vi "strobe.vi"() -> ()   [LabVIEW 2012]
uses:
  <vilib>/Platform/TimedLoop/XDataNode/timing_clust.ctl
  <vilib>/Platform/TimedLoop/XDataNode/nitl_modes.ctl
  <vilib>/Platform/TimedLoop/XDataNode/wakeup.ctl
  initialization/micron_globals.vi
  <vilib>/DAQmx/create/channels.llb/DAQmx Create Channel (CO-Pulse Generation-Frequency).vi
  <vilib>/DAQmx/configure/timing.llb/DAQmx Timing (Implicit).vi
  <vilib>/Platform/TimedLoop/XDataNode/XDataNode.xnode
  <resource>/objmgr/daqmx.rc
  <vilib>/Platform/TimedLoop/XDataNode/XDNodeRunTimeDep.lvlib
panel:
  out "Sweep duration":dbl min=0.0 step=0.001 format="%#_3p"
  out "Running":bool
  in  "Arm":bool
  out "Task":refnum<k21>
  out "Pulse rate":dbl
  in  "stop":bool
  out "Time":dbl min=0.0 step=0.001 format="%#_5p"
  in  "Offset":dbl(slide)=0.5 step=0.2 scale=-2.0..2.0 scale format="%#_2g"
  out "Phase":dbl step=5.0 format="%#.1f"
  out "Period":dbl min=0.0 step=0.001 format="%#_5p"
  in  "Center frequency":dbl(slide)=1.0 min=0.0 max=10000.0 step=1.0 scale=10.0..500.0 scale format="%#_5p"
  out "Length":dbl min=0.0 step=0.001 format="%#_5p"
  in  "Duty cycle":dbl(slide)=0.003390806681894051 scale=0.0001..0.1 scale format="%#_2g"
  in  "Sweep":cluster{"Phase":dbl, "Time":dbl}[](array[cluster])=[{"Phase"=0.0, "Time"=0.0}, {"Phase"=0.0, "Time"=0.0}] {"Time" min=0.0 step=0.001 format="%#_4p"; "Phase" step=5.0 format="%#.0f"}
  in  "Mode":bool
  in  "Source":enum16{"Auto", "Manual", "Fs"}(ring)
  # "Strobe controller"
  # "Phase"
  # "Time"
  # "Frequency"
  # "Start"
  # "End"
  # "Triggered"
  # "Continuous"
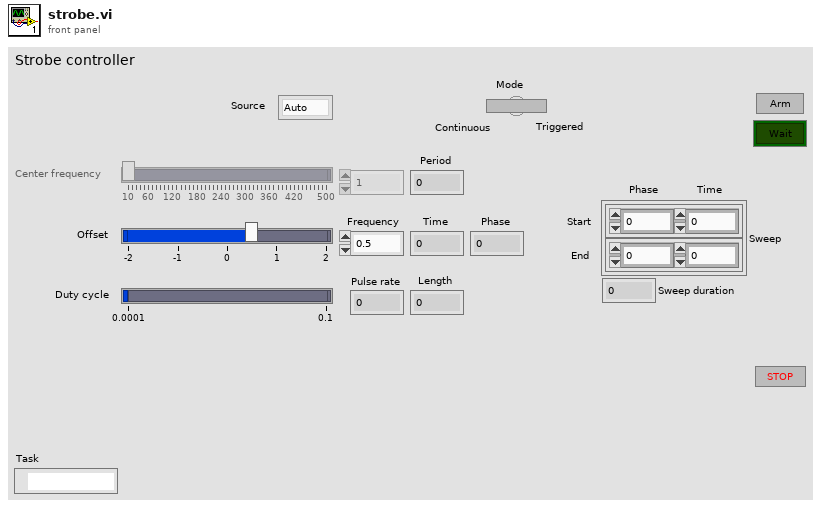
[diagram p1: front panel]
types:
  T1 = cluster{"Pulse rate":dbl, "Duty cycle":dbl, "Time":dbl, "f":i32}
  T2 = typedef "XDNodeRunTimeDep.lvlib/timing_clust.ctl" = cluster{"Expected End [f-1]":u64, "Actual End [f-1]":u64, "Finished Late? [f-1]":bool, "Expected End [i-1]":u64, "Actual End [i-1]":u64, "Finished Late? [i-1]":bool, "Expected Start [i]":u64, "Actual Start [i]":u64, "Expected Start [f]":u64, "Actual Start [f]":u64, "Source Name":string, "Structure Name":string, "Period":i64, "Deadline":i64, "Offset":i64, "Start":i64, "Priority":i32, "Timeout":i32, "Mode":T3, "Wakeup Reason":T4, "Error":errorcluster, "Source Type":string, "Secondary Source Type":string, "Global End Time":u64, "Global Start Time":u64, "Frame Duration":u64, "Iteration Duration":u64, "Assigned CPU":i32, "I/O Scan Engine Mode":u32}
  T3 = typedef "XDNodeRunTimeDep.lvlib/nitl_modes.ctl" = enum32{"No Change", "Process missed periods, maintain original phase", "Discard missed periods, maintain original phase", "Process missed periods, ignore original phase", "Discard missed periods, ignore original phase"}
  T4 = typedef "XDNodeRunTimeDep.lvlib/wakeup.ctl" = enum32{"Normal", "Aborted", "Asynchronous wakeup", "Timing source error", "Timed loop error", "Timeout"}
  T5 = typedef "micron_config.ctl" = cluster{"rt fifo":refnum<k33>, "Analog output task":refnum<k21>, "Analog output task 2":refnum<k21>, "Stimulus AO task":refnum<k21>, "Low-rate AIN task":refnum<k21>, "Pedal out task":refnum<k21>, "Pedal in task":refnum<k21>, "Loop timing source":string, "Relay out task":refnum<k21>, "Send UDP Conn":refnum<k16>, "Recv UDP Conn":refnum<k16>, "Host Addr":dbl, "I2C interface":T6, "trace_start notifier":refnum<notifier>, "trace_done notifier":refnum<notifier>, "ASAP FIFO":refnum<k33>}
  T6 = typedef "i2c_interface.ctl" = cluster{"FPGA VI Reference":T7}
  T7 = typedef "fpga_reference.ctl" = refnum<k20>
  T8 = enum8{"Enabled", "Disabled", "Disabled and Grayed Out"}
  T9 = typedef "Micron params.ctl" = cluster{"Stimulus":T10, "Goal Filter A":T12, "Mode controls":T13, "Manipulator type":enum16{"Current piezo", "Voltage piezo"}, "Manipulator calibration":T14, "Network":T16, "Goal Filter B":T12, "Cancellation":T17, "Transition time":sgl, "Estimation":T19}
  T10 = typedef "stimulus.ctl" = cluster{"Type":enum16{"Off", "Step", "Sine", "Triangle", "Arbitrary"}, "Phase":dbl, "Amplitude":sgl[], "Injection point":T11, "Closed loop":bool, "Offset":sgl[], "Tip -> world":bool, "Frequency":dbl, "Length":dbl}
  T11 = typedef "injection_point.ctl" = enum16{"Total pose", "V limiter", "Goal ", "Link position", "KF link position", "Link goal", "Link error", "Controller", "Output", "Drive", "Light"}
  T12 = typedef "goal_loop_parms.ctl" = cluster{"Speedup max":sgl, "Speedup thresh":sgl, "Speedup nonlin":sgl, "Filters":cluster{"Lower Fc":sgl, "Lower Q":sgl, "Scale factor":sgl, "Upper Fc":sgl, "Upper Q":sgl, "V limit":sgl, "V limit range":sgl}[]}
  T13 = typedef "mode_conrols.ctl" = cluster{"Hold":bool, "Cancellation":bool, "Goal filter":bool, "Trigger":bool}
  T14 = typedef "manipulator_cal.ctl" = cluster{"Tool offsets":sgl[][], "Tip light calibration":T15, "Handle light calibration":T15, "Base pivots":sgl[][], "Output pivots":sgl[][], "Length center":sgl, "Workspace height":sgl[], "Workspace diameter":sgl[], "Linearization":sgl[][], "Stack travel":sgl, "Saturation pos":sgl, "Inverse filters":cluster{"filter structure":enum32{"IIR 2nd Order", "IIR 4th Order"}, "Reverse Coefficients":dbl[], "Forward Coefficients":dbl[]}[]}
  T15 = typedef "probe_calibration.ctl" = sgl[][]
  T16 = typedef "network_params.ctl" = cluster{"Remote Host":string, "Send Status":bool, "Send Port":u16, "Recv Commands":bool, "Recv Port":u16}
  T17 = typedef "sq_control_params.ctl" = cluster{"KP":T18, "KI":sgl, "KD":T18, "Max vel":sgl, "Max acc":sgl, "Int error limit":sgl, "RCM gain":sgl, "Bypass":bool, "Degraded gain":sgl}
  T18 = typedef "decoupled_gain.ctl" = cluster{"XY":sgl, "Rxy":sgl, "Z":sgl, "Rz":sgl}
  T19 = typedef "estimation_controls.ctl" = cluster{"Link":cluster{"Measure noise":dbl[], "Process noise":dbl[], "Alt process noise":dbl[], "Innovation limit":dbl[], "Residue threshold":dbl, "Enable":bool}, "Handle":cluster{"Measure noise":dbl[], "Process noise":dbl[], "State limits":dbl[], "Innovation limit":dbl[], "Prediction Lookahead":sgl, "Enable":bool}}
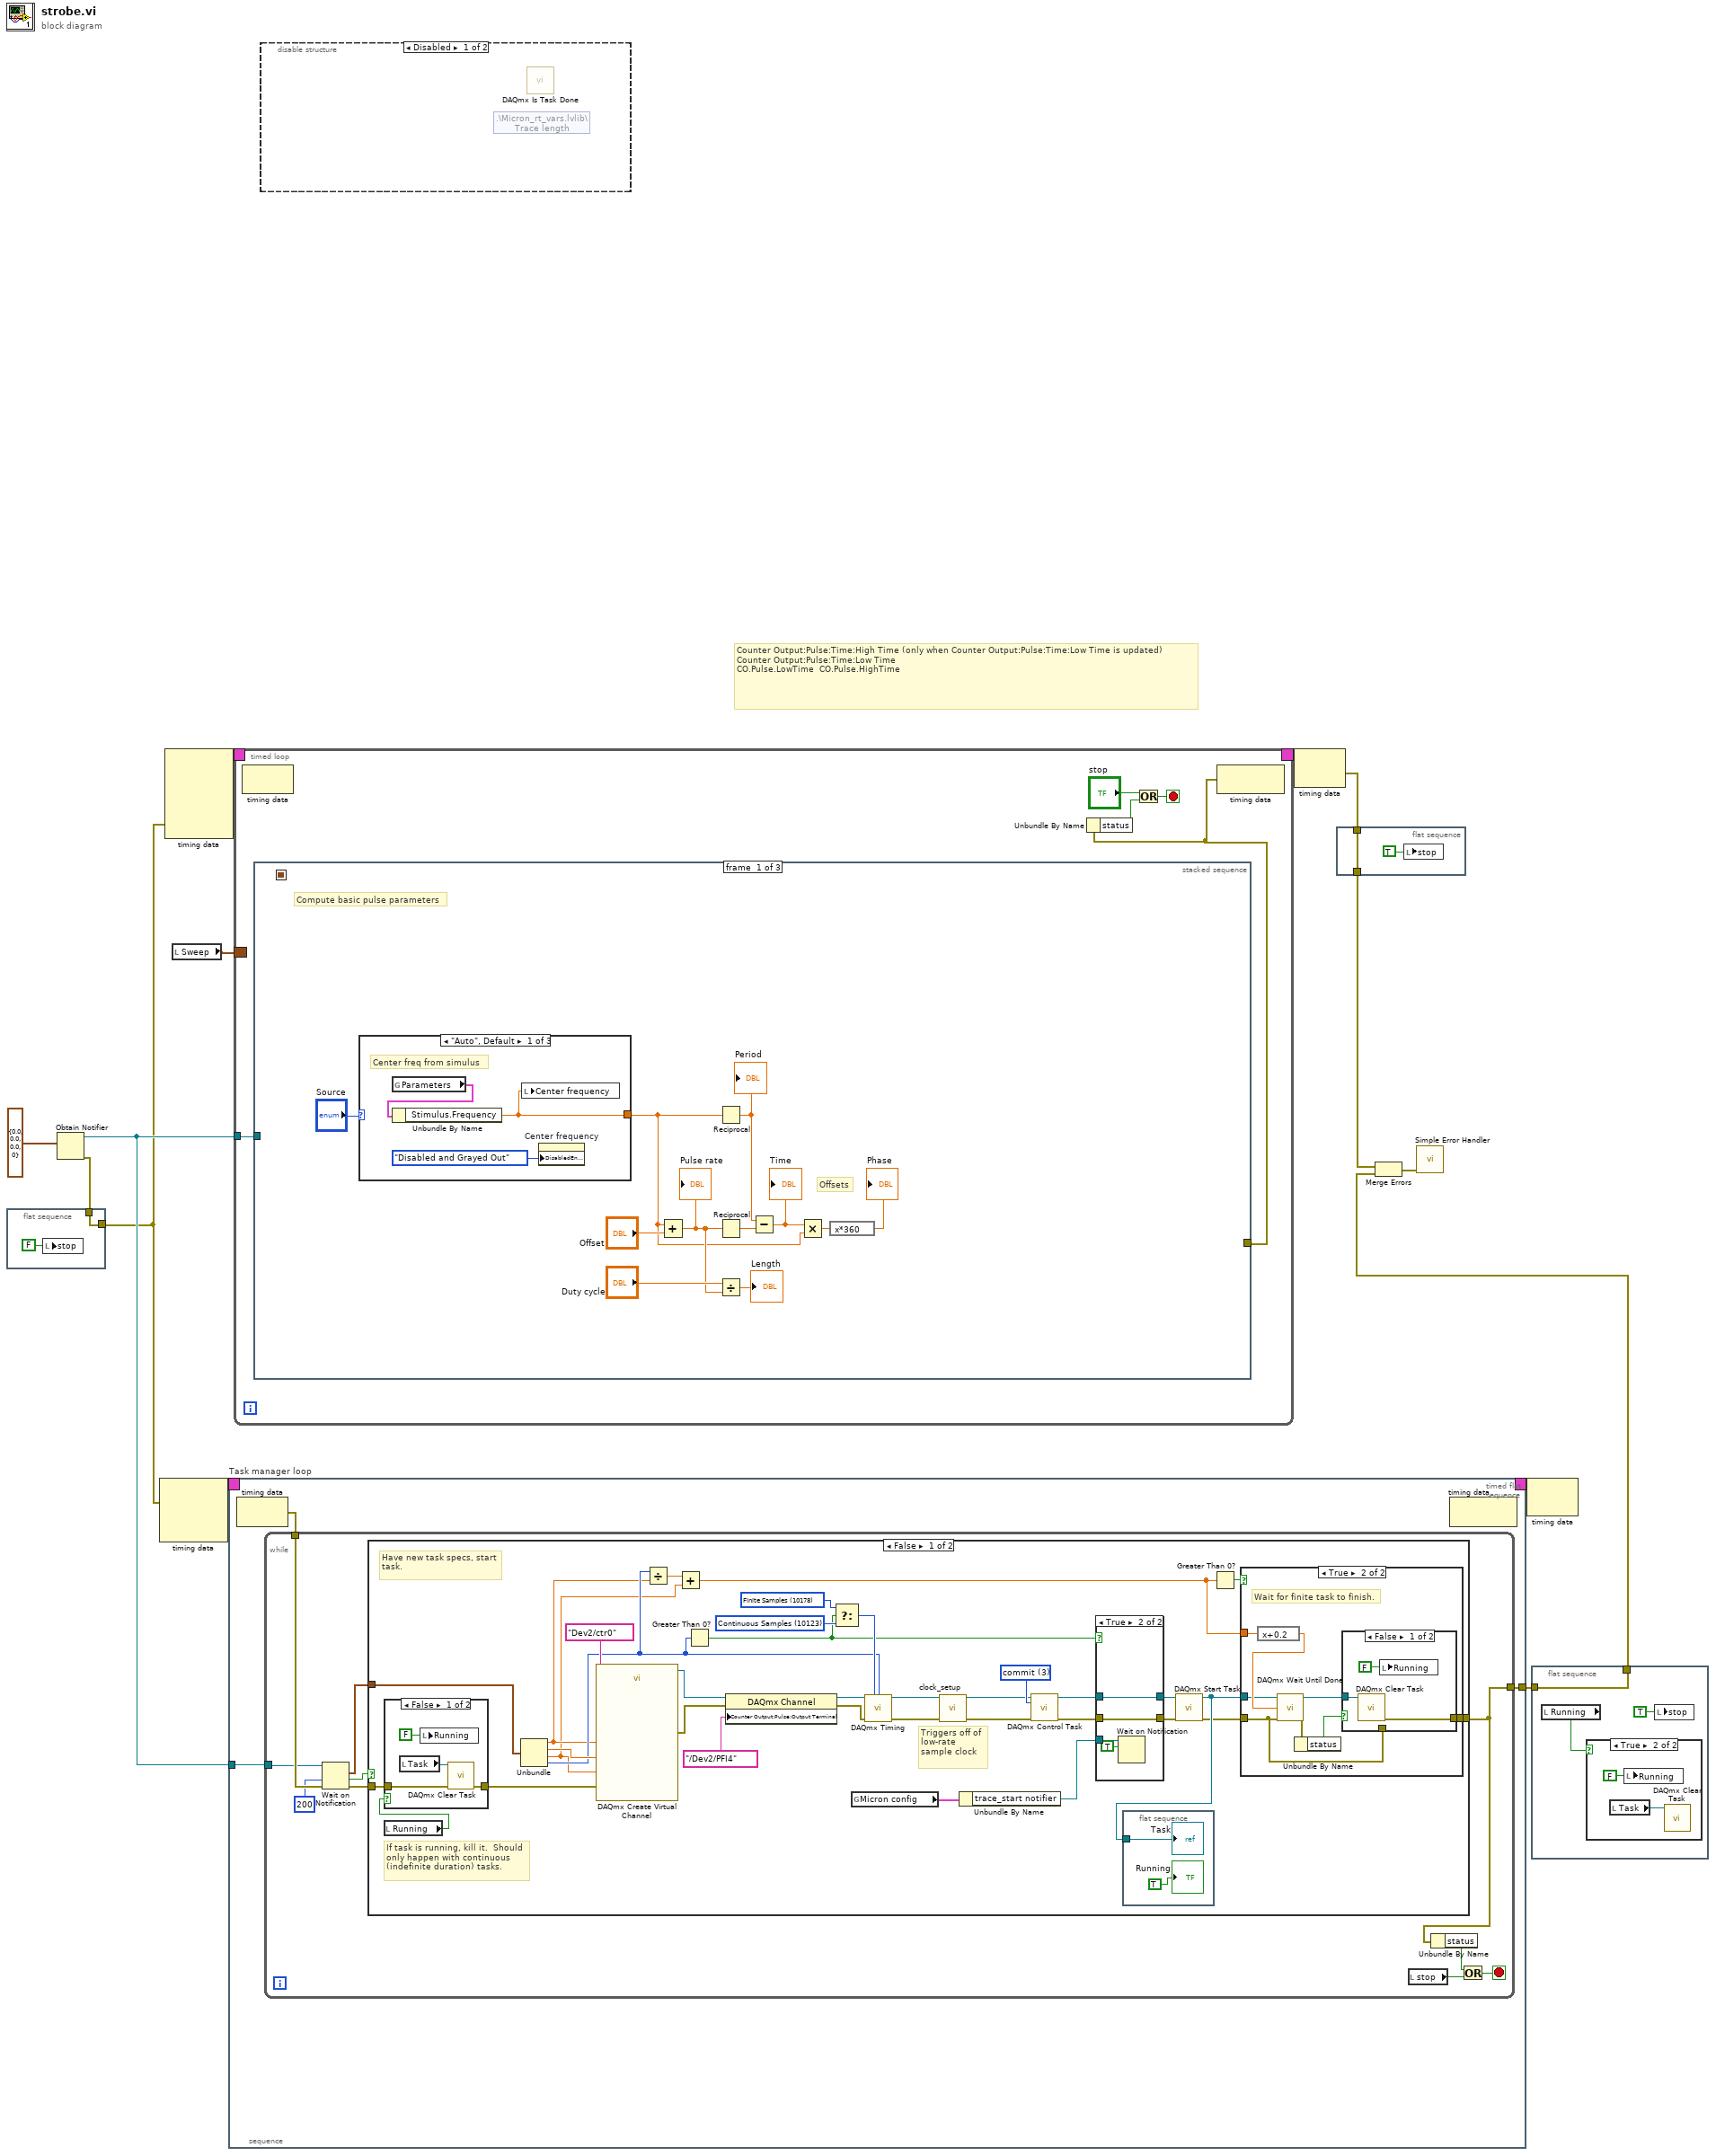
[diagram p0: block diagram]
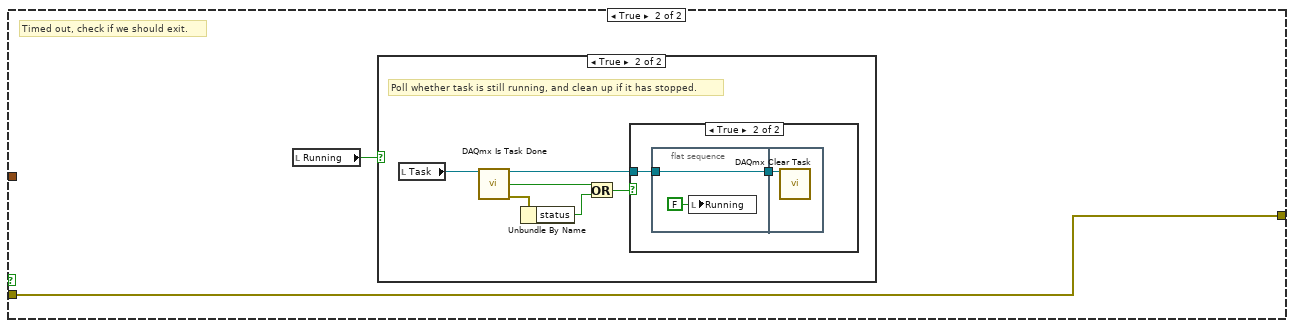
[diagram p7: hidden frame]
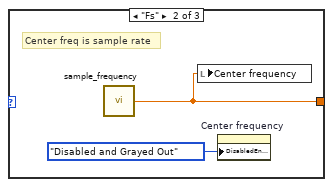
[diagram p10: hidden frame]
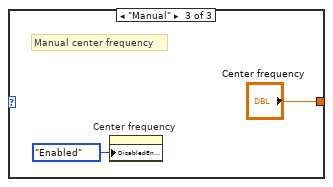
[diagram p11: hidden frame]
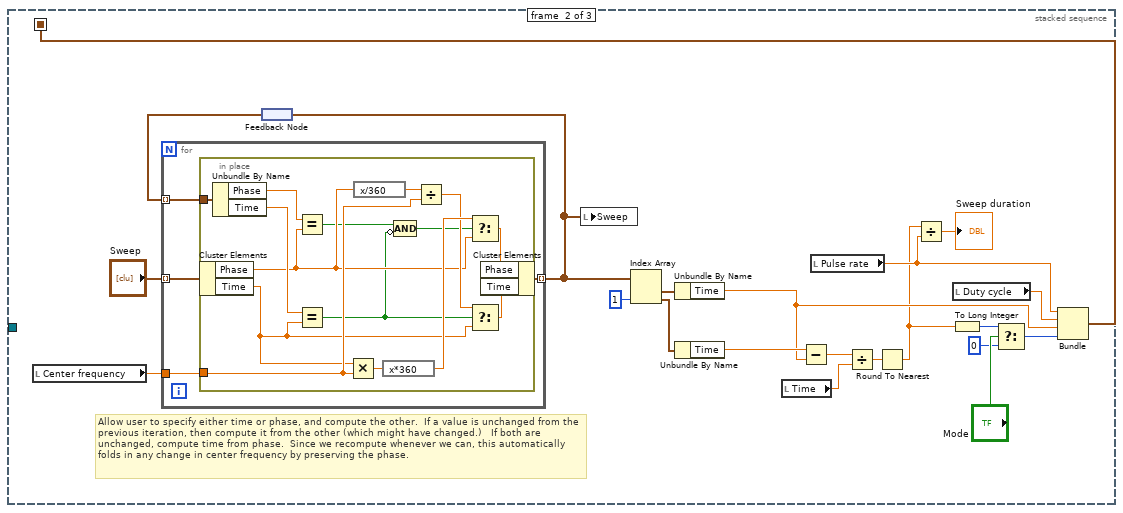
[diagram p12: hidden frame]
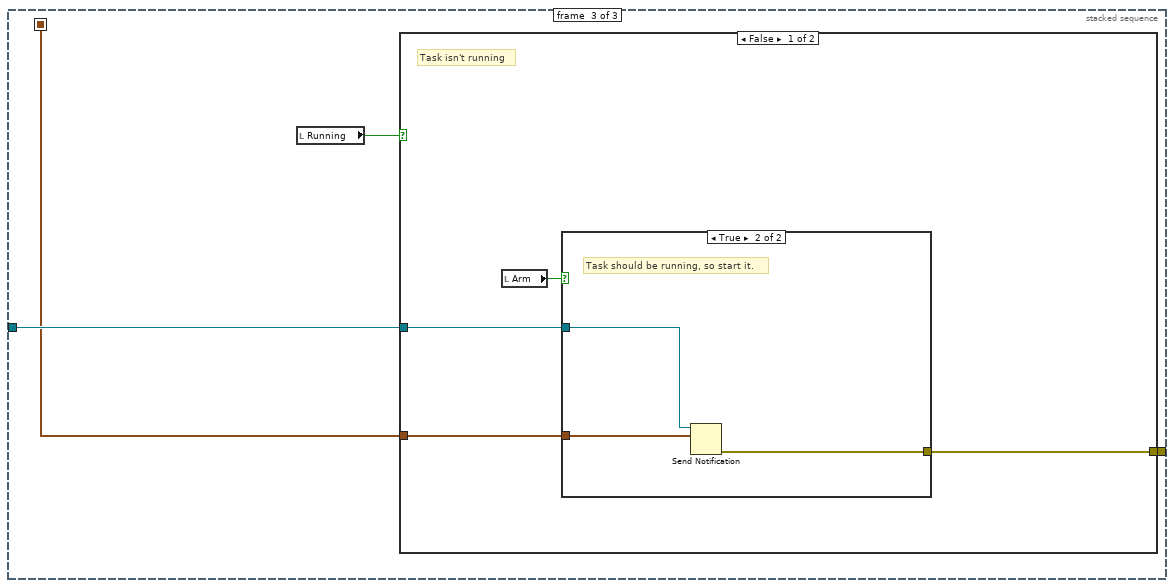
[diagram p13: hidden frame]
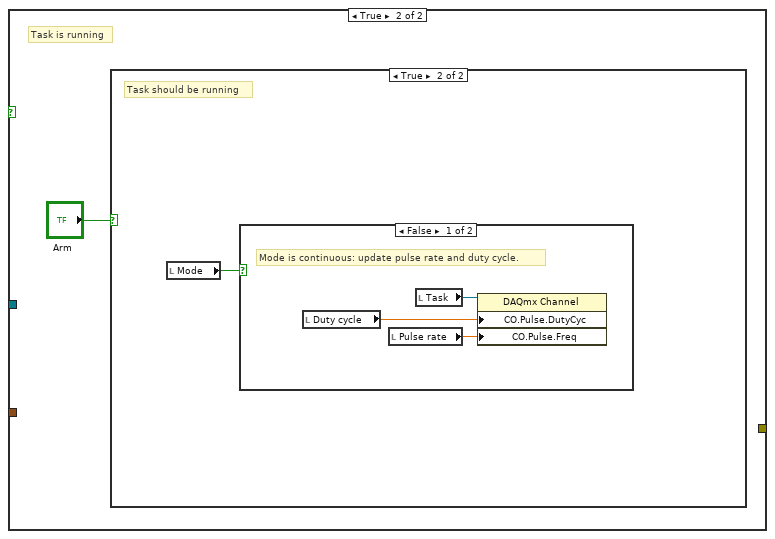
[diagram p15: hidden frame]
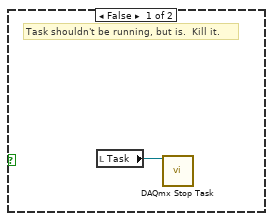
[diagram p16: hidden frame]
diagram:
  # "Counter Output:Pulse:Time:High Time (only when Counter Output:Pulse:Time:Low Time is updated) \nCounter Output:Pulse:Time:Low Time\nCO.Pulse.LowTime  CO.Pulse.HighTime"
  n1 = flat-sequence {
    tunnel: w8 -> [w16]
    tunnel: [w16] -> w7
    frame #0 {
      n2 = local write "stop"(FALSE ("stop")) -> ()
    }
  }
  n3 = Obtain Notifier(notification data type=T1 {"Pulse rate"=0.0, "Duty cycle"=0.0, "Time"=0.0, "f"=0} ("output cluster")) -> (notifier out=w10:refnum<notifier>, error out=w8:errorcluster)  [unwired: 3 in, 1 out]
  n4 = node-c288(w7) -> (w12:T2)  [unwired: 2 in]
  n5 = node-c288(w7) -> (w14:T2)  [unwired: 4 in]
  n6 = local read "Sweep"() -> (w1:cluster{"Phase":dbl, "Time":dbl}[])
  n7 = timed-sequence "Task manager loop" {
    timing: w12 -> [_]
    timing-out: [_] -> w11
    tunnel: w10 -> [w18]
    tunnel: [w17] -> w2
    n8 = timed-flat-sequence {
      tunnel: w18 -> [w20]
      tunnel: [w19] -> w17
      n9 = node-c288() -> (w21:errorcluster)  [unwired: 1 in]
      n10 = while {
        tunnel: w21 -> [w31]
        tunnel: w20 -> [w30]
        tunnel: [w22] -> w19
        stop <- w25 stop-if-true
        n11 = Wait on Notification(notifier=w30, timeout in ms (-1)=200, error in (no error)=w31) -> (notification=w29:T1, timed out?=w24:bool, error out=w28:errorcluster)  [unwired: 1 in, 1 out]
        n12 = case shown="False" w24 {
          tunnel: w29 -> [w53 _]
          tunnel: w28 -> [w41 w94]
          tunnel: [w35 w94] -> w22
          frame False {
            w50 = 10123 items=["Finite Samples"=10178, "Continuous Samples"=10123, "Hardware Timed Single Point"=12522] ("sample mode")
            w51 = 10178 items=["Finite Samples"=10178, "Continuous Samples"=10123, "Hardware Timed Single Point"=12522] ("sample mode")
            w62 = 3 items=["verify"=2, "reserve"=4, "commit"=3, "unreserve"=5, "abort"=6] ("action")
            # "If task is running, kill it.  Should\nonly happen with continuous\n(indefinite duration) tasks."
            # "Have new task specs, start task."
            # "Triggers off of low-rate sample clock"
            n13 = local read "Running"() -> (w39:bool)
            n14 = case shown="False" w39 {
              tunnel: [w85 w86] -> w40
              tunnel: w41 -> [w82 w86]
              frame False {
                n15 = local read "Task"() -> (w83:refnum<k21>)
                n16 = local write "Running"(FALSE ("Running")) -> ()
                n17 = call <vilib>:"DAQmx Clear Task.vi"("task in"=w83, "error in"=w82) -> ("error out"=w85:errorcluster)  [unwired: 13 in]
              }
              frame True {
              }
            }
            n18 = Unbundle(w53) -> ("Pulse rate"=w42:dbl, "Duty cycle"=w52:dbl, "Time"=w32:dbl, "f"=w43:i32)
            n19 = call-poly <vilib>:"DAQmx Create Virtual Channel.vi"("frequency"=w42, "duty cycle"=w52, "counter"=tag "Dev2/ctr0" ("Counter(s)"), "error in"=w40, "initial delay"=w32) -> ("task out"=w58:refnum<k21>, "error out"=w57:errorcluster)  [unwired: 4 in, 5 out]
            n20 = Divide(x=w43, y=w42) -> (x/y=w34:dbl)
            n21 = Add(x=w34, y=w32) -> (x+y=w33:dbl)
            n22 = Greater Than 0?(x=w43) -> (x > 0?=w46:bool)
            n23 = property class="DAQmx Channel"(reference=w58, error in=w57, "Counter Output:Pulse:Output Terminal"=tag "/Dev2/PFI4" ("CO.Pulse.Term")) -> (reference out=w56:refnum<k21>, error out=w55:errorcluster)
            n24 = Select(t=w51, s=w46, f=w50) -> (s? t:f=w49:i32)
            n25 = global read "micron_globals.vi" "Micron config"() -> (w45:T5)
            n26 = call-poly <vilib>:"DAQmx Timing.vi"("task/channels in"=w56, "sample mode"=w49, "samples per channel"=w43, "error in"=w55) -> ("task out"=w61:refnum<k21>, "error out"=w60:errorcluster)  [unwired: 10 out]
            n27 = call "clock_setup.vi"("task in"=w61, "error in"=w60) -> ("task out"=w48:refnum<k21>, "error out"=w47:errorcluster)  [unwired: 12 in]
            n28 = Unbundle By Name(w45) -> ("trace_start notifier"=w44:refnum<notifier>)
            n29 = call <vilib>:"DAQmx Control Task.vi"("task/channels in"=w48, "action"=w62, "error in"=w47) -> ("task out"=w65:refnum<k21>, "error out"=w63:errorcluster)  [unwired: 11 in]
            n30 = case shown="True" w46 {
              tunnel: w63 -> [w87 w92]
              tunnel: [w87 w92] -> w64
              tunnel: w65 -> [w88 w91]
              tunnel: [w88 w91] -> w66
              tunnel: w44 -> [_ w90]
              frame False {
              }
              frame True {
                n31 = Wait on Notification(notifier=w90, ignore previous (F)=TRUE) -> ()  [unwired: 2 in, 4 out]
              }
            }
            n32 = flat-sequence {
              tunnel: w37 -> [w80]
              frame #0 {
                "Task" <- w80
                "Running" <- TRUE ("Running")
              }
            }
            n33 = call <vilib>:"DAQmx Start Task.vi"("task/channels in"=w66, "error in"=w64) -> ("task out"=w37:refnum<k21>, "error out"=w36:errorcluster)  [unwired: 12 in]
            n34 = Greater Than 0?(x=w33) -> (x > 0?=w38:bool)
            n35 = case shown="True" w38 {
              tunnel: w33 -> [_ w74]
              tunnel: w37 -> [_ w72]
              tunnel: w36 -> [w67 w68]
              tunnel: [w67 w69] -> w35
              frame False {
              }
              frame True {
                # "Wait for finite task to finish."
                n36 = expression code="x+0.2"(w74) -> (w73:dbl)
                n37 = call <vilib>:"DAQmx Wait Until Done.vi"("task/channels in"=w72, "timeout (sec)"=w73, "error in"=w68) -> ("task out"=w75:refnum<k21>, "error out"=w71:errorcluster)  [unwired: 11 in]
                n38 = Unbundle By Name(w71) -> ("status"=w70:bool)
                n39 = case shown="False" w70 {
                  tunnel: w75 -> [w78 _]
                  tunnel: [w77 w79] -> w69
                  tunnel: w68 -> [_ w79]
                  frame False {
                    n40 = call <vilib>:"DAQmx Clear Task.vi"("task in"=w78) -> ("error out"=w77:errorcluster)  [unwired: 14 in]
                    n41 = local write "Running"(FALSE ("Running")) -> ()
                  }
                  frame True {
                  }
                }
              }
            }
          }
          frame True {
            # "Timed out, check if we should exit."
            n42 = local read "Running"() -> (w93:bool)
            n43 = case shown="True" w93 {
              frame False {
              }
              frame True {
                # "Poll whether task is still running, and clean up if it has stopped."
                n44 = local read "Task"() -> (w100:refnum<k21>)
                n45 = call <vilib>:"DAQmx Is Task Done.vi"("task/channels in"=w100) -> ("task out"=w95:refnum<k21>, "task done?"=w97:bool, "error out"=w99:errorcluster)  [unwired: 12 in]
                n46 = Unbundle By Name(w99) -> ("status"=w98:bool)
                n47 = Or(x=w97, y=w98) -> (x .or. y?=w96:bool)
                n48 = case shown="True" w96 {
                  tunnel: w95 -> [_ w102]
                  frame False {
                  }
                  frame True {
                    n49 = flat-sequence {
                      tunnel: w102 -> [w104]
                      tunnel: [w104] -> w101
                      tunnel: w101 -> [w105]
                      frame #0 {
                        n50 = local write "Running"(FALSE ("Running")) -> ()
                      }
                      frame #1 {
                        n51 = call <vilib>:"DAQmx Clear Task.vi"("task in"=w105) -> ()  [unwired: 14 in, 1 out]
                      }
                    }
                  }
                }
              }
            }
          }
        }
        n52 = local read "stop"() -> (w27:bool)
        n53 = Unbundle By Name(w22) -> ("status"=w26:bool)
        n54 = Or(x=w26, y=w27) -> (x .or. y?=w25:bool)
      }
      n55 = node-c288() -> ()  [unwired: 1 in, 1 out]
    }
  }
  n56 = timed-loop {
    timing: w14 -> [_]
    timing-out: [_] -> w13
    tunnel: w10 -> [w110]
    border: w1 -> [_]
    stop <- w111 stop-if-true
    n57 = node-c288() -> ()  [unwired: 1 in, 1 out]
    n58 = stacked-sequence {
      seq-local: [_ w136 _] -> [_ _ w177]
      tunnel: [_ _ w179] -> w109
      tunnel: w110 -> [_ _ w178]
      frame #0 {
        # "Compute basic pulse parameters"
        # "Offsets"
        n59 = case shown="\"Auto\", Default" "Source" {
          tunnel: [w129 w132 "Center frequency"] -> w120
          frame "Auto", Default {
            # "Center freq from simulus"
            n60 = global read "micron_globals.vi" "Parameters"() -> (w131:T9)
            n61 = Unbundle By Name(w131) -> ("Stimulus.Frequency"=w129:dbl)
            n62 = local write "Center frequency"(w129) -> ()
            n63 = property on="Center frequency" class="Slide (strict)"("DisabledEnum"=T8."Disabled and Grayed Out" ("Disabled")) -> ()  [unwired: 2 in, 2 out]
          }
          frame "Fs" {
            # "Center freq is sample rate"
            n64 = call "sample_frequency.vi"() -> ("Sample frequency"=w132:dbl)
            n65 = local write "Center frequency"(w132) -> ()
            n66 = property on="Center frequency" class="Slide (strict)"("DisabledEnum"=T8."Disabled and Grayed Out" ("Disabled")) -> ()  [unwired: 2 in, 2 out]
          }
          frame "Manual" {
            # "Manual center frequency"
            n67 = property on="Center frequency" class="Slide (strict)"("DisabledEnum"=T8."Enabled" ("Disabled")) -> ()  [unwired: 2 in, 2 out]
          }
        }
        n68 = Add(x=w120, y="Offset") -> (x+y=w124:dbl)
        "Pulse rate" <- w124
        n69 = Reciprocal(x=w120) -> (1/x=w122:dbl)
        "Period" <- w122
        n70 = Reciprocal(x=w124) -> (1/x=w123:dbl)
        n71 = Divide(x="Duty cycle", y=w124) -> (x/y=→"Length":dbl)
        n72 = Subtract(x=w122, y=w123) -> (x-y=w121:dbl)
        "Time" <- w121
        n73 = Multiply(x=w121, y=w120) -> (x*y=w119:dbl)
        n74 = expression code="x*360"(w119) -> (→"Phase":dbl)
      }
      frame #1 {
        # "Allow user to specify either time or phase, and compute the other.  If a value is unchanged from the previous iteration, then compute it from the other (which might have changed.)   If both are unchanged, compute time from phase.  Since we recompute whenever we can, this automatically folds in any change in center frequency by preserving the phase."
        n75 = local read "Center frequency"() -> (w154:dbl)
        n76 = feedback #1() -> (w155:cluster{"Phase":dbl, "Time":dbl}[])
        n77 = for {
          tunnel: "Sweep" -> [w160] mode=indexing
          tunnel: w155 -> [w159] mode=indexing
          tunnel: [w158] -> w137 mode=indexing
          tunnel: w154 -> [w157]
          n78 = in-place {
            in-place-border: w159 -> [w175]
            in-place-border: w157 -> [w167]
            n79 = in-place-cluster #2(w160) -> ("Phase"=w164:dbl, "Time"=w165:dbl)
            n80 = Unbundle By Name(w175) -> ("Phase"=w174:dbl, "Time"=w173:dbl)
            n81 = Equal?(x=w174, y=w164) -> (x = y?=w163:bool)
            n82 = Equal?(x=w173, y=w165) -> (x = y?=w162:bool)
            n83 = Multiply(x=w165, y=w167) -> (x*y=w170:dbl)
            n84 = expression code="x/360"(w164) -> (w168:dbl)
            n85 = expression code="x*360"(w170) -> (w169:dbl)
            n86 = Compound Arithmetic op=AND(w163, invert w162) -> (w161:bool)
            n87 = Divide(x=w168, y=w167) -> (x/y=w166:dbl)
            n88 = Select(t=w169, s=w161, f=w164) -> (s? t:f=w172:dbl)
            n89 = Select(t=w166, s=w162, f=w165) -> (s? t:f=w171:dbl)
            n90 = in-place-cluster #2("Phase"=w172, "Time"=w171) -> (w158:cluster{"Phase":dbl, "Time":dbl})
          }
        }
        n91 = feedback-in #1(w137) -> ()
        n92 = local write "Sweep"(w137) -> ()
        n93 = Index Array(array=w137, index #2=1 ("index")) -> (element #1=w152:cluster{"Phase":dbl, "Time":dbl}, element #2=w151:cluster{"Phase":dbl, "Time":dbl})  [unwired: 1 in]
        n94 = Unbundle By Name(w152) -> ("Time"=w144:dbl)
        n95 = Unbundle By Name(w151) -> ("Time"=w150:dbl)
        n96 = local read "Time"() -> (w143:dbl)
        n97 = Subtract(x=w150, y=w144) -> (x-y=w142:dbl)
        n98 = local read "Pulse rate"() -> (w140:dbl)
        n99 = Divide(x=w142, y=w143) -> (x/y=w141:dbl)
        n100 = Round To Nearest(number=w141) -> (nearest integer value=w139:dbl)
        n101 = Divide(x=w139, y=w140) -> (x/y=→"Sweep duration":dbl)
        n102 = To Long Integer(number=w139) -> (32bit integer=w147:i32)
        n103 = local read "Duty cycle"() -> (w149:dbl)
        n104 = Select(t=w147, s="Mode", f=0) -> (s? t:f=w145:i32)
        n105 = Bundle("Pulse rate"=w140, "Duty cycle"=w149, "Time"=w144, "f"=w145) -> (w136:T1)  [unwired: 1 in]
      }
      frame #2 {
        n106 = local read "Running"() -> (w176:bool)
        n107 = case shown="False" w176 {
          tunnel: [w182 _] -> w179
          tunnel: w178 -> [w183 _]
          tunnel: w177 -> [w181 _]
          frame False {
            # "Task isn't running"
            n108 = local read "Arm"() -> (w180:bool)
            n109 = case shown="True" w180 {
              tunnel: w183 -> [_ w186]
              tunnel: [_ w185] -> w182
              tunnel: w181 -> [_ w184]
              frame False {
                # "Task shouldn't be running, and isn't.  How about that?"
              }
              frame True {
                # "Task should be running, so start it."
                n110 = Send Notification(notification=w184, notifier=w186) -> (error out=w185:errorcluster)  [unwired: 1 in, 1 out]
              }
            }
          }
          frame True {
            # "Task is running"
            n111 = case shown="True" "Arm" {
              frame False {
                # "Task shouldn't be running, but is.  Kill it."
                n112 = local read "Task"() -> (w188:refnum<k21>)
                n113 = call <vilib>:"DAQmx Stop Task.vi"("task/channels in"=w188) -> ()  [unwired: 13 in, 2 out]
              }
              frame True {
                # "Task should be running"
                n114 = local read "Mode"() -> (w189:bool)
                n115 = case shown="False" w189 {
                  frame False {
                    # "Mode is continuous: update pulse rate and duty cycle."
                    n116 = local read "Duty cycle"() -> (w192:dbl)
                    n117 = local read "Pulse rate"() -> (w191:dbl)
                    n118 = local read "Task"() -> (w190:refnum<k21>)
                    n119 = property class="DAQmx Channel"(reference=w190, "CO.Pulse.DutyCyc"=w192, "CO.Pulse.Freq"=w191) -> ()  [unwired: 1 in, 2 out]
                  }
                  frame True {
                  }
                }
              }
            }
          }
        }
      }
    }
    n120 = Unbundle By Name(w109) -> ("status"=w113:bool)
    n121 = Or(x="stop", y=w113) -> (x .or. y?=w111:bool)
    n122 = node-c288(w109) -> ()  [unwired: 1 out]
  }
  n123 = disable-structure shown="Disabled" {
    frame Disabled {
      n124 = shared-variable ".\\Micron_rt_vars.lvlib\\Trace length"() -> ()  [unwired: 1 in, 2 out]
      n125 = call <vilib>:"DAQmx Is Task Done.vi"() -> ()  [unwired: 13 in, 3 out]
    }
    frame Enabled {
    }
  }
  n126 = node-c288(w13) -> (w6:errorcluster)
  n127 = flat-sequence {
    tunnel: w6 -> [w193]
    tunnel: [w193] -> w5
    frame #0 {
      n128 = local write "stop"(TRUE ("stop")) -> ()
    }
  }
  n129 = Merge Errors(w5, w3) -> (w4:errorcluster)
  n130 = call <vilib>:"Simple Error Handler.vi"("error in (no error)"=w4) -> ()  [unwired: 4 in, 5 out]
  n131 = node-c288(w11) -> ()  [unwired: 1 out]
  n132 = flat-sequence {
    tunnel: [w196] -> w3
    tunnel: w2 -> [w196]
    frame #0 {
      n133 = local read "Running"() -> (w195:bool)
      n134 = case shown="True" w195 {
        frame False {
        }
        frame True {
          n135 = local read "Task"() -> (w198:refnum<k21>)
          n136 = local write "Running"(FALSE ("Running")) -> ()
          n137 = call <vilib>:"DAQmx Clear Task.vi"("task in"=w198) -> ()  [unwired: 14 in, 1 out]
        }
      }
      n138 = local write "stop"(TRUE ("stop")) -> ()
    }
  }
